vi "CTR-Engine.vi"(0 "Config":T1={"enabled"=FALSE, "Hi ticks"=5, "Low ticks"=4995, "Idle state"=10214, "Delay ticks"=0} {"Idle state" items=["High"=10192, "Low"=10214]; "Low ticks" max=1}, 2 "action":T2=enum."Configure", 9 "Sync task in":refnum<k21>, 11 "error in (no error)":errorcluster) -> (15 "error out":errorcluster)   [LabVIEW 2020]
uses:
  Typedefs/CTR-Action.ctl
  Typedefs/CTR-Config.ctl
  AIDI/Typedefs/AIDI-Action.ctl
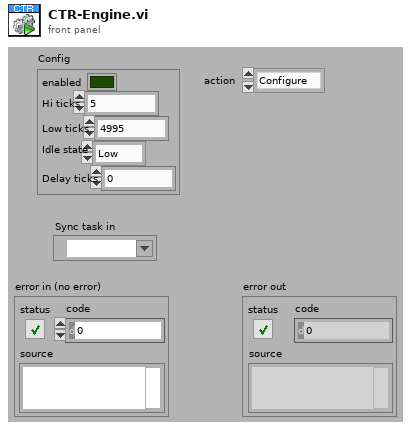
[diagram p1: front panel]
types:
  T1 = typedef "CTR-Config.ctl" = cluster{"enabled":bool, "Hi ticks":u32, "Low ticks":u32, "Idle state":i32, "Delay ticks":u32}
  T2 = typedef "CTR-Action.ctl" = enum16{"Clear", "Configure", "Initialize", "Init & Start", "Start", "Clean up"}
  T3 = typedef "AIDI-Action.ctl" = enum16{"Configure", "Initialize", "Start", "Read", "Clean up", "Init & Start", "Config & Test", "Position", "Skip"}
  T4 = typedef "CTR-Task Specification.ctl" = cluster{"task":string}
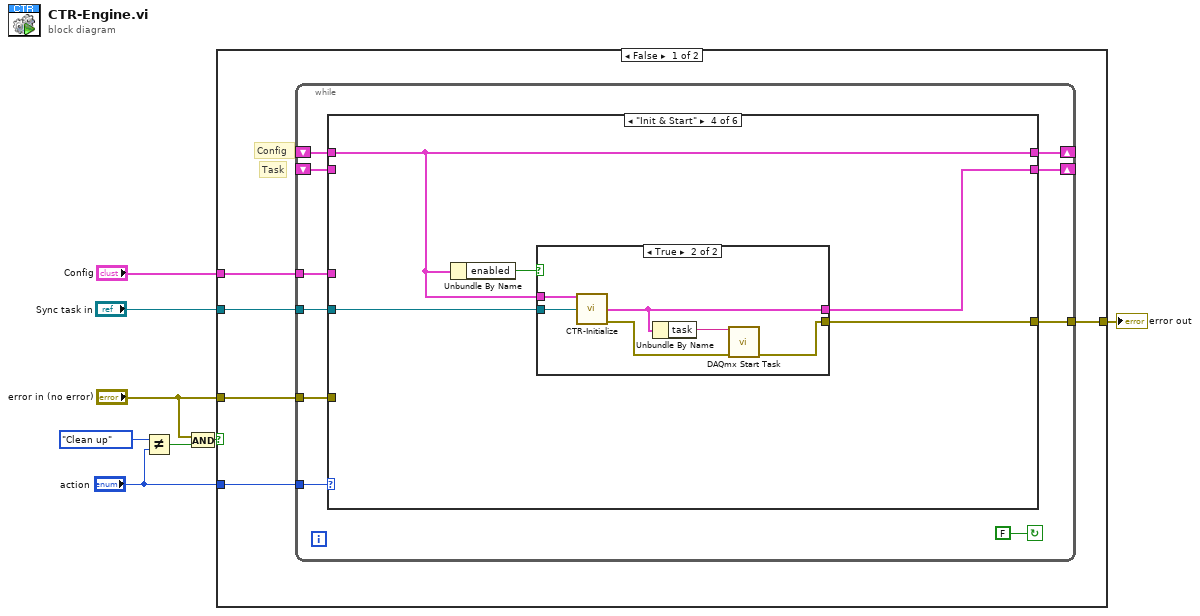
[diagram p0: block diagram]
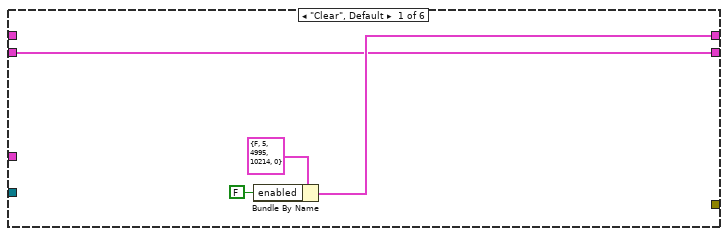
[diagram p2: hidden frame]
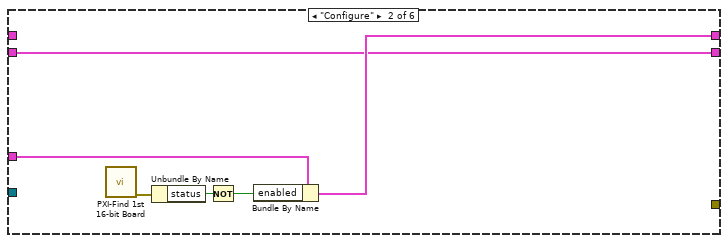
[diagram p3: hidden frame]
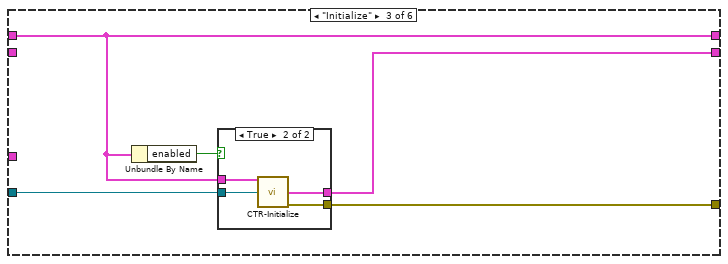
[diagram p4: hidden frame]
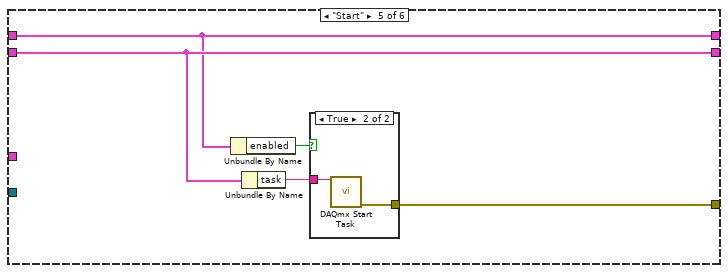
[diagram p7: hidden frame]
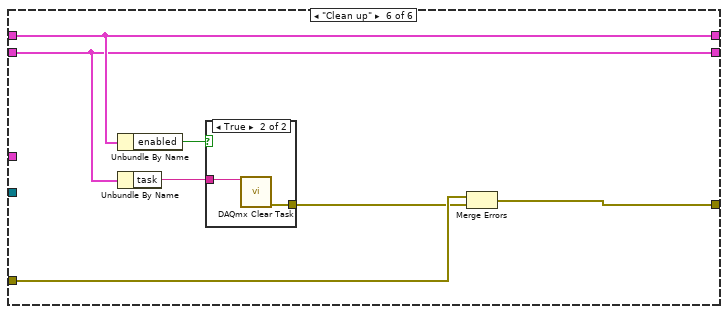
[diagram p9: hidden frame]
diagram:
  n1 = Not Equal?(x=AIDI-Action."Clean up", y="action") -> (x != y?=w4:bool)
  n2 = And(x="error in (no error)", y=w4) -> (x .and. y?=w5:bool)
  n3 = case shown="False" w5 {
    tunnel: "action" -> [w13 _]
    tunnel: [w12 w70] -> w8
    tunnel: "error in (no error)" -> [w11 w70]
    tunnel: "Sync task in" -> [w10 _]
    tunnel: "Config" -> [w9 _]
    frame False {
      # "Config"
      # "Task"
      n4 = while {
        shift-right: [w19] -> _
        shift-left: _ -> [w15]
        tunnel: [w22] -> w12
        shift-right: [w21] -> _
        shift-left: _ -> [w20]
        tunnel: w13 -> [w23]
        tunnel: w11 -> [w17]
        tunnel: w10 -> [w16]
        tunnel: w9 -> [w14]
        stop <- FALSE continue-if-true
        n5 = case shown="\"Init & Start\"" w23 {
          tunnel: [_ _ w37 w46 w56 w67] -> w22
          tunnel: [w25 w33 w35 w44 w55 w65] -> w21
          tunnel: w20 -> [_ _ w35 w44 w55 w65]
          tunnel: [w24 w32 w36 w45 w58 w63] -> w19
          tunnel: w17 -> [_ _ _ _ _ w66]
          tunnel: w16 -> [_ _ w34 w43 _ _]
          tunnel: w15 -> [w24 w32 _ _ w58 w63]
          tunnel: w14 -> [_ w28 _ _ _ _]
          frame "Clear", Default {
            n6 = Bundle By Name(cluster=T1 {"enabled"=FALSE, "Hi ticks"=5, "Low ticks"=4995, "Idle state"=10214, "Delay ticks"=0} ("Config"), "enabled"=FALSE) -> (w25:T1)
          }
          frame "Configure" {
            n7 = call "PXI-Find 1st 16-bit Board.vi"() -> ("error out"=w30:errorcluster)  [unwired: 9 in, 2 out]
            n8 = Unbundle By Name(w30) -> ("status"=w31:bool)
            n9 = Not(x=w31) -> (.not. x?=w29:bool)
            n10 = Bundle By Name(cluster=w28, "enabled"=w29) -> (w33:T1)
          }
          frame "Initialize" {
            n11 = Unbundle By Name(w35) -> ("enabled"=w38:bool)
            n12 = case shown="True" w38 {
              tunnel: [_ w42] -> w37
              tunnel: [_ w41] -> w36
              tunnel: w35 -> [_ w40]
              tunnel: w34 -> [_ w39]
              frame False {
              }
              frame True {
                n13 = call "CTR-Initialize.vi"("Config"=w40, "task"=w39) -> ("Counter Task"=w41:T4, "error out"=w42:errorcluster)  [unwired: 12 in]
              }
            }
          }
          frame "Init & Start" {
            n14 = Unbundle By Name(w44) -> ("enabled"=w47:bool)
            n15 = case shown="True" w47 {
              tunnel: [_ w50] -> w46
              tunnel: [_ w49] -> w45
              tunnel: w44 -> [_ w53]
              tunnel: w43 -> [_ w52]
              frame False {
              }
              frame True {
                n16 = call "CTR-Initialize.vi"("Config"=w53, "task"=w52) -> ("Counter Task"=w49:T4, "error out"=w51:errorcluster)  [unwired: 12 in]
                n17 = Unbundle By Name(w49) -> ("task"=w48:string)
                n18 = call <vilib>:"DAQmx Start Task.vi"("task/channels in"=w48, "error in"=w51) -> ("error out"=w50:errorcluster)  [unwired: 12 in, 1 out]
              }
            }
          }
          frame "Start" {
            n19 = Unbundle By Name(w55) -> ("enabled"=w54:bool)
            n20 = Unbundle By Name(w58) -> ("task"=w57:string)
            n21 = case shown="True" w54 {
              tunnel: w57 -> [_ w60]
              tunnel: [_ w59] -> w56
              frame False {
              }
              frame True {
                n22 = call <vilib>:"DAQmx Start Task.vi"("task/channels in"=w60) -> ("error out"=w59:errorcluster)  [unwired: 13 in, 1 out]
              }
            }
          }
          frame "Clean up" {
            n23 = Unbundle By Name(w65) -> ("enabled"=w64:bool)
            n24 = Unbundle By Name(w63) -> ("task"=w62:string)
            n25 = case shown="True" w64 {
              tunnel: w62 -> [_ w69]
              tunnel: [_ w68] -> w61
              frame False {
              }
              frame True {
                n26 = call <vilib>:"DAQmx Clear Task.vi"("task in"=w69) -> ("error out"=w68:errorcluster)  [unwired: 14 in]
              }
            }
            n27 = Merge Errors(w66, w61) -> (w67:errorcluster)
          }
        }
      }
    }
    frame True {
    }
  }
  "error out" <- w8
